vi "Ack Response.vi"(8 "error in (no error)":errorcluster, 9 "Original TCP Payload":T1, 11 "TCPMessageAPI in":refnum<class "TCPMessageAPI.lvclass">) -> (0 "error out":errorcluster, 3 "TCPMessageAPI out":refnum<class "TCPMessageAPI.lvclass">)   [LabVIEW 2020, in "Vecto.lvlib" / "TCPMessageAPI.lvclass"]
uses:
  TCPMessageAPI.lvclass
  proto/TcpPayload/Data.ctl
  proto/AckNackResult/Enumeration.ctl
  proto/AckNackResult/AckNackResult.lvlib
  proto/TcpPayload/TcpPayload.lvlib
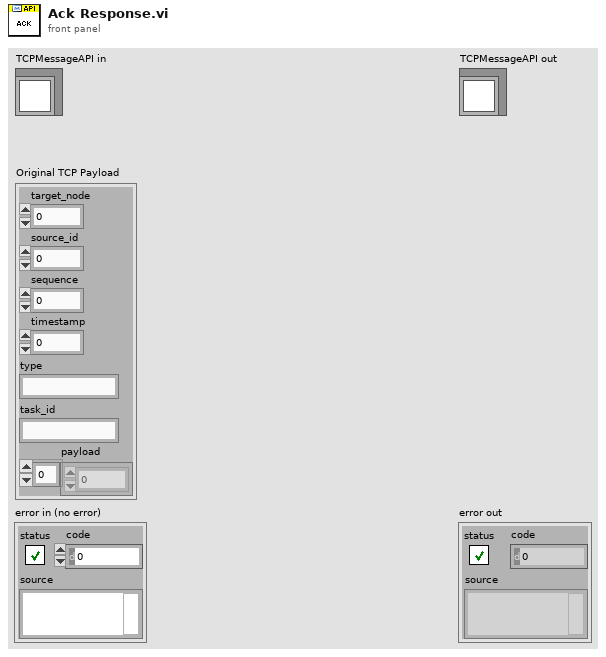
[diagram p1: front panel]
types:
  T1 = typedef "TcpPayload.lvlib/Data.ctl" = cluster{"target_node":u32, "source_id":u32, "sequence":u32, "timestamp":i64, "type":string, "task_id":string, "payload":u8[]}
  T2 = typedef "AckNackResult.lvlib/Enumeration.ctl" = enum16{"RESULT_PAYLOAD_ERROR", "RESULT_UNEXPECTED_TYPE", "RESULT_EXPIRED", "RESULT_OUTOFSEQUENCE", "RESULT_DISALLOWED", "RESULT_INVALIDTASK", "RESULT_INVALIDTARGET", "RESULT_UNKNOWN", "RESULT_ACK"}
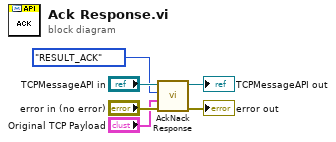
[diagram p0: block diagram]
diagram:
  n1 = call "AckNack Response.vi"("error in (no error)"="error in (no error)", "Original TCP Payload"="Original TCP Payload", "Result"=Enumeration."RESULT_ACK", "TCPMessageService in"="TCPMessageAPI in") -> ("error out"=→"error out":errorcluster, "TCPMessageService out"=→"TCPMessageAPI out":refnum<class "TCPMessageAPI.lvclass">)  [unwired: 6 in]
